vi "Populate Font ComboBox.vi"(8 "error in":errorcluster, 9 "Font in":string, 11 "CmbBox Refnum":refnum<vi>) -> (0 "error out":errorcluster, 1 "Font out":string)   [LabVIEW 2020]
uses:
  vi.lib/LabVIEW Icon API/lv_icon/lv_icon.lvlib
  <vilib>/registry/registry.llb/Registry SAM.ctl
  ed04b51d-df56-4900-9d1c-7b9855d0d70f.vi
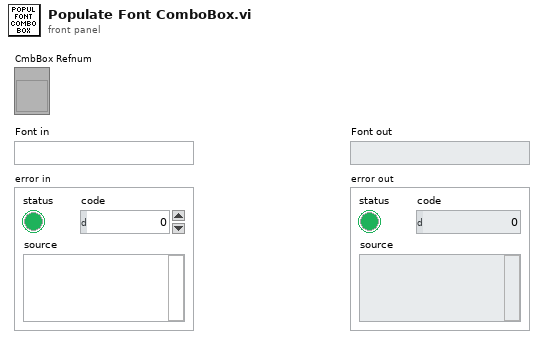
[diagram p1: front panel]
types:
  T1 = typedef "Registry SAM.ctl" = enum32{"KEY_QUERY_VALUE", "KEY_SET_VALUE", "KEY_CREATE_SUB_KEY", "KEY_ENUMERATE_SUB_KEYS", "KEY_NOTIFY", "KEY_CREATE_LINK", "KEY_READ", "KEY_WRITE", "KEY_ALL_ACCESS", "KEY_READ | KEY_WRITE"}
  T2 = typedef "Registry refnum.ctl" = refnum<k1>
  T3 = cluster{"numValues":i32, "maxValueNameLen":i32, "maxValueDataLen":i32}
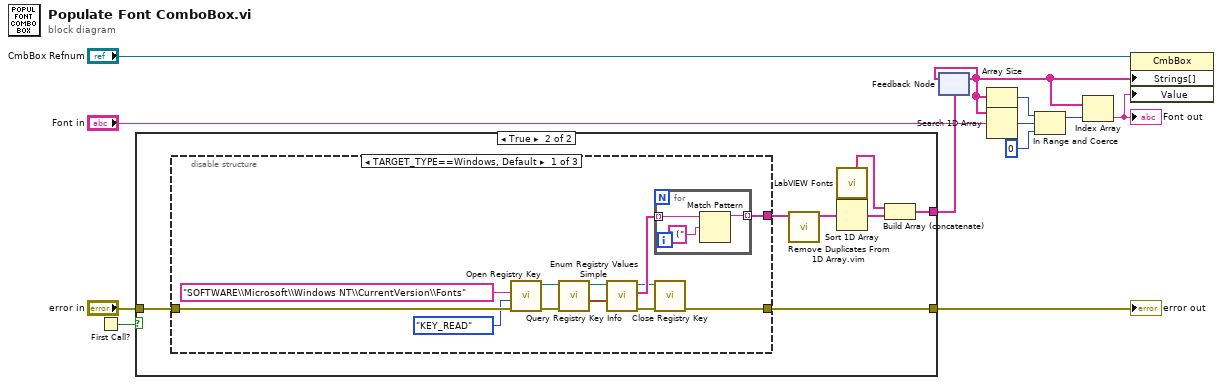
[diagram p0: block diagram]
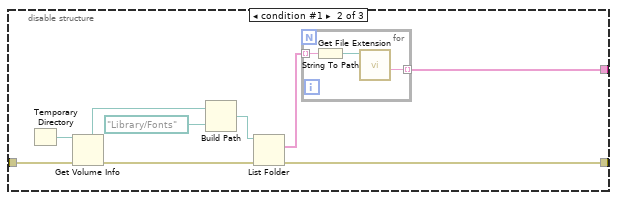
[diagram p3: hidden frame]
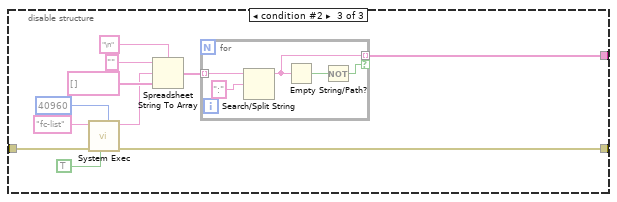
[diagram p4: hidden frame]
diagram:
  n1 = First Call?() -> (First Call?: T/F=w3:bool)
  n2 = case shown="True" w3 {
    tunnel: "error in" -> [w13 w20]
    tunnel: [w13 w19] -> w11
    tunnel: [_ w16] -> w4
    frame False {
    }
    frame True {
      n3 = disable-structure shown="TARGET_TYPE==Windows, Default" {
        disable-tunnel: w20 -> [w30 w43 w58]
        disable-tunnel: [w29 w42 w57] -> w19
        disable-tunnel: [w21 w36 w48] -> w15
        frame condition #0 (active) {
          n4 = call <vilib>:"Open Registry Key.vi"("error in (no error)"=w30, "security access mask (KEY_READ | KEY_WRITE)"=Registry_SAM."KEY_READ", "subkey"="SOFTWARE\\Microsoft\\Windows NT\\CurrentVersion\\Fonts") -> ("error out"=w31:errorcluster, "refnum out"=w24:T2)  [unwired: 1 in, 6 out]
          n5 = call <vilib>:"Query Registry Key Info.vi"("error in (no error)"=w31, "refnum"=w24) -> ("value info"=w25:T3, "refnum out"=w26:T2)  [unwired: 8 out]
          n6 = call <vilib>:"Enum Registry Values Simple.vi"("value info"=w25, "refnum"=w26) -> ("error out"=w32:errorcluster, "values"=w28:string[], "refnum out"=w27:T2)  [unwired: 2 in, 5 out]
          n7 = for {
            tunnel: w28 -> [w35] mode=indexing
            tunnel: [w33] -> w21 mode=indexing
            n8 = Match Pattern(string=w35, regular expression=" (") -> (before substring=w33:string)  [unwired: 4 out]
          }
          n9 = call <vilib>:"Close Registry Key.vi"("error in (no error)"=w32, "refnum"=w27) -> ("error out"=w29:errorcluster)  [unwired: 5 out]
        }
        frame condition #1 {
          n10 = Temporary Directory() -> (w41:path)
          n11 = Get Volume Info(8:w43, 11:w41) -> (0:w44:errorcluster, 5:w40:path)  [unwired: 4 out]
          n12 = Build Path(base path=w40, name or relative path=path "Library/Fonts") -> (appended path=w39:path)
          n13 = List Folder(path=w39, error in=w44) -> (filenames=w38:string[], error out=w42:errorcluster)  [unwired: 4 out]
          n14 = for {
            tunnel: w38 -> [w47] mode=indexing
            tunnel: [w45] -> w36 mode=indexing
            n15 = String To Path(string=w47) -> (path=w46:path)
            n16 = call <vilib>:"Get File Extension.vi"("file"=w46) -> ("filename without extension"=w45:string)  [unwired: 1 in, 9 out]
          }
        }
        frame condition #2 {
          n17 = call <vilib>:"System Exec.vi"("expected output size  (4096)"=u32 40960, "run minimized? (F)"=TRUE, "error in (no error)"=w58, "command line"="fc-list") -> ("error out"=w57:errorcluster, "standard output"=w49:string)  [unwired: 3 in, 3 out]
          n18 = Spreadsheet String To Array(delimiter (Tab)="\n", format string="", spreadsheet string=w49, array type (2D Dbl)=string[] []) -> (array=w50:string[])
          n19 = for {
            tunnel: w50 -> [w63] mode=indexing
            tunnel: [w61] -> w48 mode=indexing if=w59
            n20 = Search/Split String(string=w63, search string/char (-)=":") -> (substring before match=w61:string)  [unwired: 3 out]
            n21 = Empty String/Path?(string/path=w61) -> (empty?=w60:bool)
            n22 = Not(x=w60) -> (.not. x?=w59:bool)
          }
        }
      }
      n23 = call "Remove Duplicates From 1D Array.vim"("array"=w15) -> ("array with duplicates removed"=w14:string[])  [unwired: 10 in]
      n24 = call "LabVIEW Fonts.vi"() -> ("Additional Fonts"=w18:string[])  [unwired: 1 in, 10 out]
      n25 = Sort 1D Array(array=w14) -> (sorted array=w17:string[])
      n26 = Build Array (concatenate)(w18, w17) -> (w16:string[])
    }
  }
  "error out" <- w11
  n27 = feedback #1(w4) -> (w5:string[])
  n28 = feedback-in #1(w5) -> ()
  n29 = Array Size(array=w5) -> (size(s)=w7:i32)
  n30 = Search 1D Array(1D array=w5, element="Font in") -> (index of element=w10:i32)  [unwired: 1 out]
  n31 = In Range and Coerce(upper limit=w7, x=w10, lower limit=0 ("x")) -> (coerced(x)=w8:i32)  [unwired: 1 out]
  n32 = Index Array(array=w5, index=w8) -> (element=w1:string)
  "Font out" <- w1
  n33 = property class="CmbBox"(reference="CmbBox Refnum", "Strings[]"=w5, "Value"=w1) -> ()  [unwired: 1 in, 2 out]
